vi "SEA-9811_ReceiverAndTransmitter_RT.vi"() -> ()   [LabVIEW 2012]
doc: "This example demonstrates the SEA 9811 receiver and transmitter in normal mode. Transmitter and receiver can be used simultaneously. In order to receive transmitter data connect the transmitter line with the receiver lines at module's front connector. Please also refer to the FPGA VI.\n\n<B>Prerequisites:</B>\n1. CompactRIO system (LabVIEW 2011)\n2. SEA 9811\n3. In order to receive sent data: adapter that connects transmitter line with Receiver line(s) (not included with the SEa 9811 module).\n\n<B>Instructions:</B>\n1. Run the VI\n2. Enter data to be written in <B>Tx Data</B> and write it pressing the corresponding button\n3. Observe thet all 8 channels indicate that receiver FIFOs are NOT empty*\n4. Observe that the sent data is shown in <B>Channel's Rx Data</B>*\n5. Stop the VI\n\n* only if an adequate adatper connects the transmitter lines with the receiver line(s).\n\nCopyright (c) 2013 S.E.A. Datentechnik GmbH, Germany"
uses:
  <vilib>/rvi/interface/nirviReadWriteControl/nirviReadWriteControl.xnode
  <vilib>/rvi/interface/nirviCloseFPGA/nirviCloseFPGA.xnode
  <vilib>/rvi/interface/nirviMethod/nirviMethod.xnode
  SubVIs/SEA-9811_ReceiverAndTransmitter_RCR.ctl
  SubVIs/SEA-9811_ReceiverAndTransmitter_TCR.ctl
  <vilib>/rvi/errors/niLvFpgaAdjustHostInterfaceError.vi
  <vilib>/rvi/errors/niLvFpgaMergeErrorWithErrorCode.vi
  <vilib>/rvi/interface/nirviOpenFPGA/nirviOpenFPGA.xnode
  <vilib>/rvi/interface/Simulation/niFpgaSimulationCallBeginRW.vi
  <vilib>/FPGAPlugInAG/Dynamic/niLvFpga_ReadFifo_Dynamic.vi
  <vilib>/FPGAPlugInAG/Dynamic/niLvFpga_Reset_Dynamic.vi
  <vilib>/FPGAPlugInAG/Dynamic/niLvFpga_Run_Dynamic.vi
  NiFpgaLv.dll
  <vilib>/Utility/error.llb/Error Cluster From Error Code.vi
  SEA-9811_ReceiverAndTransmitter_FPGA.vi
  <vilib>/FPGAPlugInAG/cRIO-9104/niLvFpga_Open_cRIO-9104.vi
  <vilib>/rvi/interface/common/dynamic/niFpgaDynamicAddResources.vi
  <vilib>/FPGAPlugInAG/Dynamic/niLvFpga_Close_Dynamic.vi
  SubVIs/SEA-9811_ReceiverAndTransmitter_RSR.ctl
  SubVIs/SEA-9811_ReceiverAndTransmitter_TSR.ctl
panel:
  in  "Rx Channel Number (0..7)":u8
  out "Transmitter Status Register (TSR)":T1={"TSR0: undefined"=FALSE, "TSR1: undefined"=FALSE, "TSR2: undefined"=FALSE, "TSR3: Transmitter FIFO empty?"=TRUE, "TSR4: Transmitter FIFO contains at least (TRUE)/less than (FALSE) 16 words"=FALSE, "TSR5: Transmitter FIFO full? (contains 32 words)"=FALSE, "TSR6: undefined"=FALSE, "TSR7: undefined"=FALSE}
  out "Receiver Status Register (RSR)":T2={"RSR0: FIFO channel 0 empty"=TRUE, "RSR1: FIFO channel 1 empty"=TRUE, "RSR2: FIFO channel 2 empty"=TRUE, "RSR3: FIFO channel 3 empty"=TRUE, "RSR4: FIFO channel 4 empty"=TRUE, "RSR5: FIFO channel 5 empty"=TRUE, "RSR6: FIFO channel 6 empty"=TRUE, "RSR7: FIFO channel 7 empty"=TRUE, "RSR8: FIFO channel 0 full"=FALSE, "RSR9: FIFO channel 1 full"=FALSE, "RSR10: FIFO channel 2 full"=FALSE, "RSR11: FIFO channel 3 full"=FALSE, "RSR12: FIFO channel 4 full"=FALSE, "RSR13: FIFO channel 5 full"=FALSE, "RSR14: FIFO channel 6 full"=FALSE, "RSR15: FIFO channel 7 full"=FALSE}
  in  "Rx Label Filter":T3
  in  "Transmit Cyclic":bool
  in  "Transmit Once":bool
  in  "Tx Data":u32 format="%08x"
  out "Channel's Rx Data":u32[](array[numeric]) format="%.0x"
  out "DMA Overflow":bool
  in  "stop":bool
  # "Please refer to VI description for instructions!"
  # "Receiver"
  # "Transmitter"
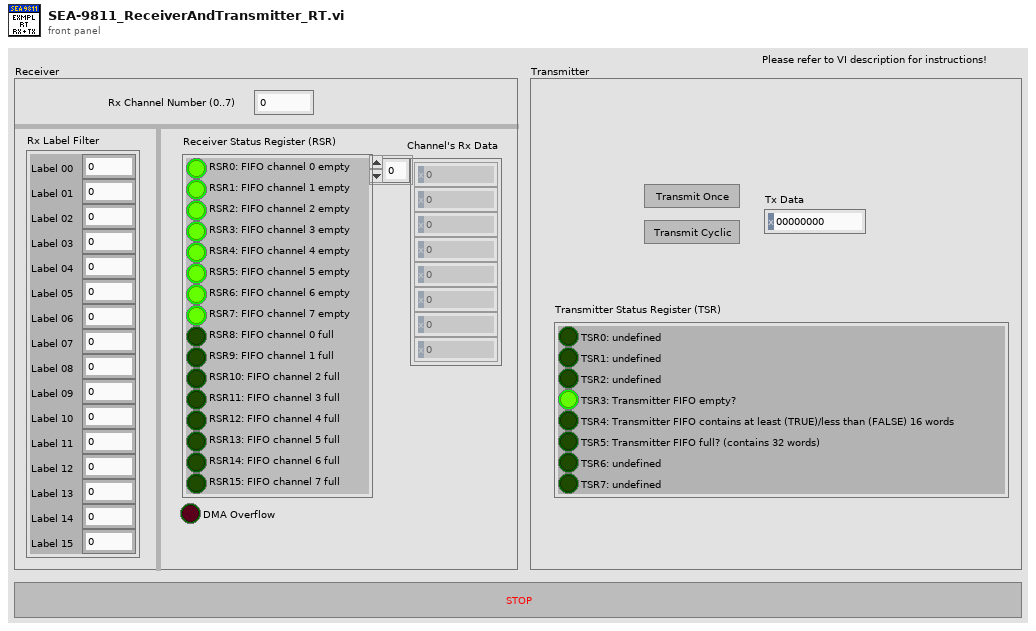
[diagram p1: front panel]
types:
  T1 = typedef "SEA-9811_ReceiverAndTransmitter_TSR.ctl" = cluster{"TSR0: undefined":bool, "TSR1: undefined":bool, "TSR2: undefined":bool, "TSR3: Transmitter FIFO empty?":bool, "TSR4: Transmitter FIFO contains at least (TRUE)/less than (FALSE) 16 words":bool, "TSR5: Transmitter FIFO full? (contains 32 words)":bool, "TSR6: undefined":bool, "TSR7: undefined":bool}
  T2 = typedef "SEA-9811_ReceiverAndTransmitter_RSR.ctl" = cluster{"RSR0: FIFO channel 0 empty":bool, "RSR1: FIFO channel 1 empty":bool, "RSR2: FIFO channel 2 empty":bool, "RSR3: FIFO channel 3 empty":bool, "RSR4: FIFO channel 4 empty":bool, "RSR5: FIFO channel 5 empty":bool, "RSR6: FIFO channel 6 empty":bool, "RSR7: FIFO channel 7 empty":bool, "RSR8: FIFO channel 0 full":bool, "RSR9: FIFO channel 1 full":bool, "RSR10: FIFO channel 2 full":bool, "RSR11: FIFO channel 3 full":bool, "RSR12: FIFO channel 4 full":bool, "RSR13: FIFO channel 5 full":bool, "RSR14: FIFO channel 6 full":bool, "RSR15: FIFO channel 7 full":bool}
  T3 = cluster{"Label 00":u8, "Label 01":u8, "Label 02":u8, "Label 03":u8, "Label 04":u8, "Label 05":u8, "Label 06":u8, "Label 07":u8, "Label 08":u8, "Label 09":u8, "Label 10":u8, "Label 11":u8, "Label 12":u8, "Label 13":u8, "Label 14":u8, "Label 15":u8}
  T4 = typedef "SEA-9811_ReceiverAndTransmitter_RCR.ctl" = cluster{"RCR0: Data rate = ARINC 429 High-Speed (0) or Low-Speed (1)":bool, "RCR1: not used":bool, "RCR2: Label recognition for this channel enabled (1) or disabled (0)":bool, "RCR3: Receiver channel disabled (1) or enabled (0)":bool, "RCR4: Odd parity check for this channel enabled (1) or disabled (0":bool, "RCR5: Receiver normal operation (1) or loopback mode (0)":bool, "RCR6: Receiver Decoder disabled (0) or enabled (1) -> ARINC bits 10 and 9 must match RCR7 and RCR8":bool, "RCR7: If receiver decoder is enabled (RCR6=1), the ARINC bit 10 must match this bit":bool, "RCR8: If receiver decoder is enabled (RCR6=1), the ARINC bit 9 must match this bit":bool, "RCR9: Label bit order for this channel non-reversed (1) or reversed (0)":bool, "RCR10: not used":bool, "RCR11: not used":bool, "RCR12: not used":bool, "RCR13: not used":bool, "RCR14: not used":bool, "RCR15: not used":bool}
  T5 = typedef "SEA-9811_ReceiverAndTransmitter_TCR.ctl" = cluster{"TCR0: not used":bool, "TCR1: not used":bool, "TCR2: not used":bool, "TCR3: Transmitter Parity Bit Enable: 32nd bit is parity (1) or data (0)":bool, "TCR4: not used":bool, "TCR5: not used":bool, "TCR6: not used":bool, "TCR7: not used":bool, "TCR8: not used":bool, "TCR9: Transmitter Parity Select: odd parity (0) or even parity (1)":bool, "TCR10: Transmitter Data Rate: ARINC 429 high-speed (0) or low-speed (1)":bool, "TCR11: ARINC Label Bit Order: label bit order reversed (0) or not reversed (1)":bool, "TCR12: Disable Line Driver: normal operation (0) or transmitter disabled (1)":bool, "TCR13: Tansmit whenever data is available in FIFO (1) or only start by instruction \"Enable Transmission\" (0)":bool, "TCR14: not used":bool, "TCR15: not used":bool}
  T6 = cluster{"Boolean array[0]":bool, "Boolean array[1]":bool, "Boolean array[2]":bool, "Boolean array[3]":bool, "Boolean array[4]":bool, "Boolean array[5]":bool, "Boolean array[6]":bool, "Boolean array[7]":bool, "Boolean array[8]":bool, "Boolean array[9]":bool, "Boolean array[10]":bool, "Boolean array[11]":bool, "Boolean array[12]":bool, "Boolean array[13]":bool, "Boolean array[14]":bool, "Boolean array[15]":bool}
  T7 = cluster{"Boolean array[0]":bool, "Boolean array[1]":bool, "Boolean array[2]":bool, "Boolean array[3]":bool, "Boolean array[4]":bool, "Boolean array[5]":bool, "Boolean array[6]":bool, "Boolean array[7]":bool}
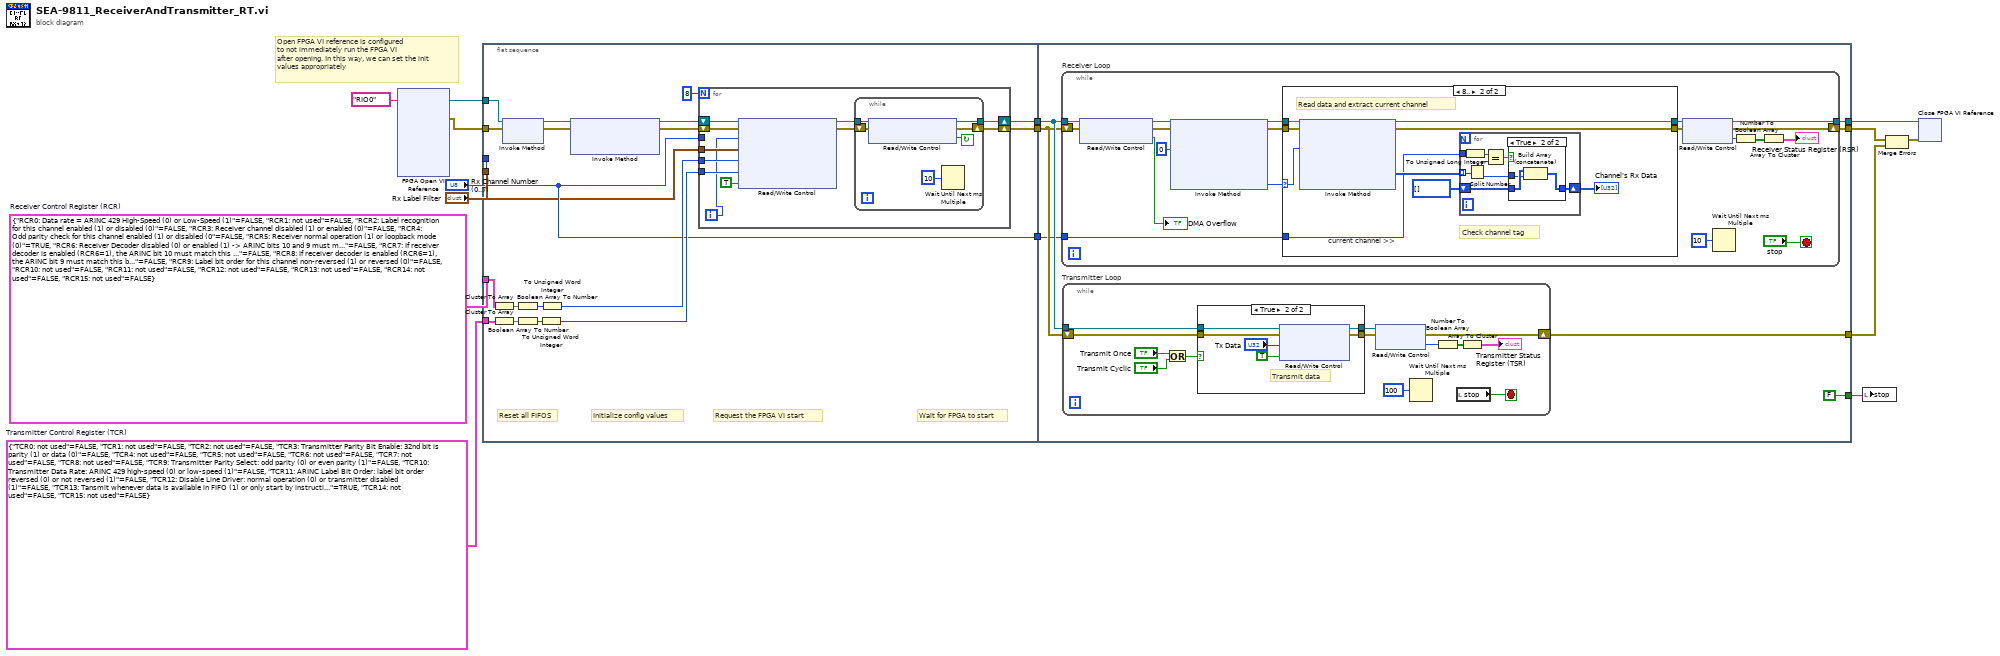
[diagram p0: block diagram]
diagram:
  w11 = T4 {"RCR0: Data rate = ARINC 429 High-Speed (0) or Low-Speed (1)"=FALSE, "RCR1: not used"=FALSE, "RCR2: Label recognition for this channel enabled (1) or disabled (0)"=FALSE, "RCR3: Receiver channel disabled (1) or enabled (0)"=FALSE, "RCR4: Odd parity check for this channel enabled (1) or disabled (0"=FALSE, "RCR5: Receiver normal operation (1) or loopback mode (0)"=TRUE, "RCR6: Receiver Decoder disabled (0) or enabled (1) -> ARINC bits 10 and 9 must match RCR7 and RCR8"=FALSE, "RCR7: If receiver decoder is enabled (RCR6=1), the ARINC bit 10 must match this bit"=FALSE, "RCR8: If receiver decoder is enabled (RCR6=1), the ARINC bit 9 must match this bit"=FALSE, "RCR9: Label bit order for this channel non-reversed (1) or reversed (0)"=FALSE, "RCR10: not used"=FALSE, "RCR11: not used"=FALSE, "RCR12: not used"=FALSE, "RCR13: not used"=FALSE, "RCR14: not used"=FALSE, "RCR15: not used"=FALSE}  # Receiver Control Register (RCR)
  w10 = T5 {"TCR0: not used"=FALSE, "TCR1: not used"=FALSE, "TCR2: not used"=FALSE, "TCR3: Transmitter Parity Bit Enable: 32nd bit is parity (1) or data (0)"=FALSE, "TCR4: not used"=FALSE, "TCR5: not used"=FALSE, "TCR6: not used"=FALSE, "TCR7: not used"=FALSE, "TCR8: not used"=FALSE, "TCR9: Transmitter Parity Select: odd parity (0) or even parity (1)"=FALSE, "TCR10: Transmitter Data Rate: ARINC 429 high-speed (0) or low-speed (1)"=FALSE, "TCR11: ARINC Label Bit Order: label bit order reversed (0) or not reversed (1)"=FALSE, "TCR12: Disable Line Driver: normal operation (0) or transmitter disabled (1)"=FALSE, "TCR13: Tansmit whenever data is available in FIFO (1) or only start by instruction \"Enable Transmission\" (0)"=TRUE, "TCR14: not used"=FALSE, "TCR15: not used"=FALSE}  # Transmitter Control Register (TCR)
  # "Open FPGA VI reference is configured\nto not immediately run the FPGA VI\nafter opening. In this way, we can set the init\nvalues appropriately"
  n1 = xnode "FPGA Open VI Reference"("resource name"=tag "RIO0") -> ("FPGA VI Reference Out"=w2:refnum<k20>, "error out"=w1:errorcluster)  [unwired: 1 in]
  n2 = flat-sequence {
    tunnel: [w17] -> w8
    tunnel: [w18] -> w7
    tunnel: [w20] -> w6
    tunnel: w1 -> [w25]
    tunnel: w2 -> [w26]
    tunnel: w10 -> [w29]
    tunnel: w11 -> [w34]
    tunnel: "Rx Channel Number (0..7)" -> [w20]
    tunnel: "Rx Label Filter" -> [w19]
    tunnel: [w58] -> w15
    tunnel: w8 -> [w56]
    tunnel: w7 -> [w57]
    tunnel: [w55] -> w9
    tunnel: [w54] -> w5
    tunnel: w6 -> [w53]
    tunnel: [FALSE ("stop")] -> w4
    frame #0 {
      # "Initialize config values"
      # "Reset all FIFOS"
      # "Wait for FPGA to start"
      # "Request the FPGA VI start"
      n3 = Cluster To Array(cluster=w34) -> (array=w33:bool[])
      n4 = Cluster To Array(cluster=w29) -> (array=w30:bool[])
      n5 = xnode "Invoke Method"("FPGA VI Reference In"=w26, "error in"=w25) -> ("FPGA VI Reference Out"=w24:refnum<k20>, "error out"=w22:errorcluster)
      n6 = Boolean Array To Number(Boolean array=w33) -> (number=w32:u32)
      n7 = Boolean Array To Number(Boolean array=w30) -> (number=w31:u32)
      n8 = To Unsigned Word Integer(number=w31) -> (unsigned 16bit integer=w27:u16)
      n9 = To Unsigned Word Integer(number=w32) -> (unsigned 16bit integer=w28:u16)
      n10 = xnode "Invoke Method"("FPGA VI Reference In"=w24, "error in"=w22) -> ("FPGA VI Reference Out"=w23:refnum<k20>, "error out"=w21:errorcluster)  [unwired: 1 in]
      n11 = for {
        N: 8 -> [_]
        tunnel: w28 -> [w45]
        tunnel: w27 -> [w44]
        tunnel: w20 -> [_]
        tunnel: w19 -> [w41]
        shift-right: [w36] -> w17
        shift-left: w21 -> [w42]
        shift-right: [w37] -> w18
        shift-left: w23 -> [w43]
        i -> [w35]
        n12 = xnode "Read/Write Control"("FPGA VI Reference In"=w43, "error in"=w42, "Rx Channel Number"=w35, "Rx Label Filter"=w41, "Rx Config Data (RCR)"=w45, "Tx Config Data (TCR)"=w44, "Configure channel"=TRUE) -> ("FPGA VI Reference Out"=w39:refnum<k20>, "error out"=w38:errorcluster)
        n13 = while {
          tunnel: w39 -> [w51]
          tunnel: [w47] -> w37
          shift-right: [w46] -> w36
          shift-left: w38 -> [w50]
          stop <- w49 continue-if-true
          n14 = xnode "Read/Write Control"("FPGA VI Reference In"=w51, "error in"=w50) -> ("FPGA VI Reference Out"=w47:refnum<k20>, "error out"=w46:errorcluster, "Configure channel"=w49:bool)
          n15 = Wait Until Next ms Multiple(millisecond multiple=u32 10) -> ()  [unwired: 1 out]
        }
      }
    }
    frame #1 {
      n16 = while "Receiver Loop" {
        tunnel: w57 -> [w83]
        tunnel: [w96] -> w58
        shift-right: [w95] -> w54
        shift-left: w56 -> [w82]
        tunnel: w53 -> [w80]
        stop <- "stop" stop-if-true
        n17 = xnode "Read/Write Control"("FPGA VI Reference In"=w83, "error in"=w82) -> ("FPGA VI Reference Out"=w85:refnum<k20>, "error out"=w84:errorcluster, "DMA Overflow"=→"DMA Overflow":bool)
        n18 = xnode "Invoke Method"("FPGA VI Reference In"=w85, "error in"=w84, "Number of Elements"=u32 0) -> ("FPGA VI Reference Out"=w91:refnum<k20>, "error out"=w90:errorcluster, "Elements Remaining"=w81:u32)  [unwired: 1 in, 1 out]
        n19 = case shown="8.." w81 {
          selector: w81 -> [_ w105]
          tunnel: w91 -> [w100 w109]
          tunnel: w90 -> [w99 w108]
          tunnel: [w100 w107] -> w88
          tunnel: [w99 w106] -> w87
          tunnel: w80 -> [_ w101]
          frame Default {
            # "not enough data to read"
          }
          frame 8.. {
            # "Check channel tag"
            # "Read data and extract current channel"
            # "current channel >>"
            n20 = xnode "Invoke Method"("FPGA VI Reference In"=w109, "error in"=w108, "Number of Elements"=w105) -> ("FPGA VI Reference Out"=w107:refnum<k20>, "error out"=w106:errorcluster, "Data"=w104:u64[])  [unwired: 1 in, 1 out]
            n21 = for {
              tunnel: w104 -> [w117] mode=indexing
              shift-right: [w111] -> w102
              shift-left: u32[] [] -> [w112]
              tunnel: w101 -> [w115]
              n22 = To Unsigned Long Integer(number=w115) -> (unsigned 32bit integer=w110:u32)
              n23 = Split Number(x=w117) -> (hi(x)=w116:u32, lo(x)=w113:u32)
              n24 = Equal?(x=w110, y=w116) -> (x = y?=w114:bool)
              n25 = case shown="True" w114 {
                tunnel: w113 -> [_ w120]
                tunnel: w112 -> [w118 w121]
                tunnel: [w118 w119] -> w111
                frame False {
                }
                frame True {
                  n26 = Build Array (concatenate)(w121, w120) -> (w119:u32[])
                }
              }
            }
            "Channel's Rx Data" <- w102
          }
        }
        n27 = xnode "Read/Write Control"("FPGA VI Reference In"=w88, "error in"=w87) -> ("FPGA VI Reference Out"=w96:refnum<k20>, "error out"=w95:errorcluster, "Rx Status"=w94:u16)
        n28 = Wait Until Next ms Multiple(millisecond multiple=u32 10) -> ()  [unwired: 1 out]
        n29 = Number To Boolean Array(number=w94) -> (Boolean array=w93:bool[])
        n30 = Array To Cluster(array=w93) -> (cluster=→"Receiver Status Register (RSR)":T6)
      }
      n31 = while "Transmitter Loop" {
        tunnel: w57 -> [w70]
        shift-right: [w62] -> w55
        shift-left: w56 -> [w69]
        stop <- w71 stop-if-true
        n32 = Or(x="Transmit Once", y="Transmit Cyclic") -> (x .or. y?=w68:bool)
        n33 = case shown="True" w68 {
          tunnel: w70 -> [w73 w79]
          tunnel: w69 -> [w72 w78]
          tunnel: [w73 w75] -> w64
          tunnel: [w72 w74] -> w63
          frame False {
          }
          frame True {
            # "Transmit data"
            n34 = xnode "Read/Write Control"("FPGA VI Reference In"=w79, "error in"=w78, "Tx Data"="Tx Data", "Transmit Data"=TRUE ("Trsanmit Data")) -> ("FPGA VI Reference Out"=w75:refnum<k20>, "error out"=w74:errorcluster)
          }
        }
        n35 = xnode "Read/Write Control"("FPGA VI Reference In"=w64, "error in"=w63) -> ("error out"=w62:errorcluster, "Tx Status"=w61:u8)  [unwired: 1 out]
        n36 = Wait Until Next ms Multiple(millisecond multiple=u32 100) -> ()  [unwired: 1 out]
        n37 = Number To Boolean Array(number=w61) -> (Boolean array=w60:bool[])
        n38 = local read "stop"() -> (w71:bool)
        n39 = Array To Cluster(array=w60) -> (cluster=→"Transmitter Status Register (TSR)":T7)
      }
    }
  }
  n40 = local write "stop"(w4) -> ()
  n41 = Merge Errors(w5, w9) -> (w14:errorcluster)
  n42 = xnode "Close FPGA VI Reference"("FPGA VI Reference In"=w15, "error in"=w14) -> ()  [unwired: 1 out]
